vi "MB Exception Code to Error Message.vi"(11 "Exception Code":u8 format="%.0x") -> (3 "Error Message":string)   [LabVIEW 2010]
panel:
  in  "Error Messages":string[](array[string])=["", "Illegal function", "Illegal data address", "Illegal data value", "failure in associated device", "Acknowledge", "Busy, rejected message", "NAK- Negative acknowledge"]
  # "VI Name: MB Exception Code to Error Message.vi\nPurpose: Creates the error message corresponding\n                to the exception code."
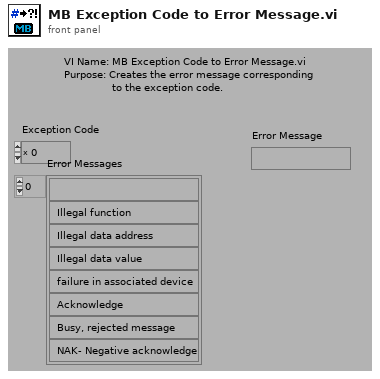
[diagram p1: front panel]
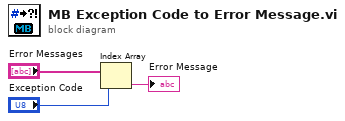
[diagram p0: block diagram]
diagram:
  n1 = Index Array(array="Error Messages", index="Exception Code") -> (element=→"Error Message":string)
